vi "Velocity Conversion.vi"(11 "Velocity (ft/s)":dbl) -> (3 "Velocity (ticks/ds)":dbl)   [LabVIEW 2020]
doc: "dimensional analysis: feet per second --> ticks per decisecond (falcon units)"
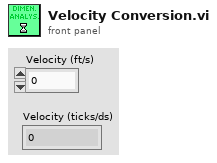
[diagram p1: front panel]
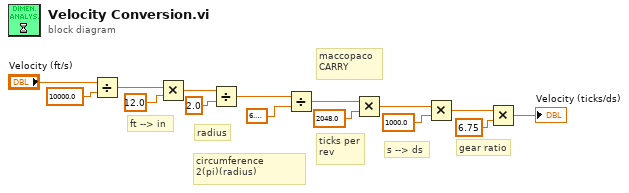
[diagram p0: block diagram]
diagram:
  # "s --> ds"
  # "circumference\n2(pi)(radius)"
  # "ticks per\nrev"
  # "ft --> in"
  # "radius"
  # "gear ratio"
  # "maccopaco\nCARRY"
  n1 = Divide(x="Velocity (ft/s)", y=10000.0) -> (x/y=w13:dbl)
  n2 = Multiply(x=w13, y=12.0) -> (x*y=w11:dbl)
  n3 = Divide(x=w11, y=2.0) -> (x/y=w9:dbl)
  n4 = Divide(x=w9, y=6.283185307179586) -> (x/y=w8:dbl)
  n5 = Multiply(x=w8, y=2048.0) -> (x*y=w6:dbl)
  n6 = Multiply(x=w6, y=1000.0) -> (x*y=w4:dbl)
  n7 = Multiply(x=w4, y=6.75) -> (x*y=→"Velocity (ticks/ds)":dbl)
